vi "DrivePath.vi"() -> ()   [LabVIEW 2018]
uses:
  Dawgma Programming Library/Controls/PurePursuit/PathFileData.ctl
  Dawgma Programming Library/Controls/PurePursuit/RobotNeededPathData.ctl
  Framework/Robot Global Data.vi
panel:
  in  "NoWait":bool
  in  "Index":i32
  in  "Path":string
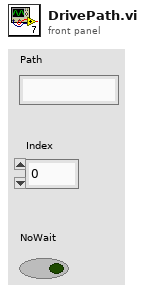
[diagram p1: front panel]
types:
  T1 = typedef "PathFileData.ctl" = cluster{"RobotNeeded":T2, "Meta":cluster{"Path (px)":cluster{i32, i32}[], "RobotWidth":dbl, "RobotLength":dbl, "CenterOfRotYOffset":dbl, "Roundedness":dbl, "StartingPositionPreset":u32}}
  T2 = typedef "RobotNeededPathData.ctl" = cluster{"Path":cluster{dbl, dbl}[], "MaxVel":dbl, "MaxAccel":dbl, "Backwards?":bool, "PointSpacing":dbl, "LookaheadDist":dbl, "Speed/Curve":dbl, "SlowDistanceAtEnd":dbl, "SlowSpeed":dbl, "MaxDeAccel":dbl}
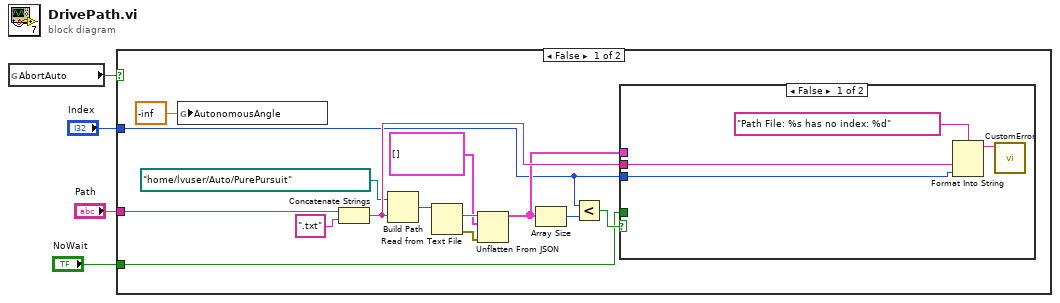
[diagram p0: block diagram]
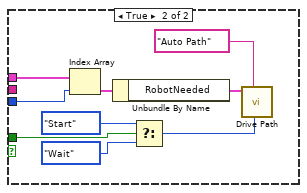
[diagram p2: hidden frame]
diagram:
  n1 = global read "Robot Global Data.vi" "AbortAuto"() -> (w4:bool)
  n2 = case shown="False" w4 {
    tunnel: "Index" -> [w7 _]
    tunnel: "NoWait" -> [w6 _]
    tunnel: "Path" -> [w5 _]
    frame False {
      n3 = global write "Robot Global Data.vi" "AutonomousAngle"(-inf ("AutonomousAngle")) -> ()
      n4 = Concatenate Strings(w5, ".txt" ("string")) -> (w18:string)
      n5 = Build Path(base path=path "/home/lvuser/Auto/PurePursuit", name or relative path=w18) -> (appended path=w14:path)
      n6 = Read from Text File(file (use dialog)=w14) -> (text=w13:string, error out=w12:errorcluster)  [unwired: 3 in, 2 out]
      n7 = Unflatten From JSON(JSON string=w13, type and defaults=T1[] [], error in (no error)=w12) -> (value=w15:T1[])  [unwired: 4 in, 1 out]
      n8 = Array Size(array=w15) -> (size(s)=w16:i32)
      n9 = Less?(x=w7, y=w16) -> (x < y?=w17:bool)
      n10 = case shown="False" w17 {
        tunnel: w7 -> [w20 w31]
        tunnel: w6 -> [_ w27]
        tunnel: w15 -> [_ w23]
        tunnel: w18 -> [w19 _]
        frame False {
          n11 = Format Into String(format string="Path File: %s has no index: %d", w19, w20) -> (resulting string=w22:string)  [unwired: 2 in, 1 out]
          n12 = call "CustomError.vi"("String"=w22) -> ()  [unwired: 10 in, 1 out]
        }
        frame True {
          n13 = Index Array(array=w23, index=w31) -> (element=w30:T1)
          n14 = Unbundle By Name(w30) -> ("RobotNeeded"=w29:T2)
          n15 = Select(t=enum16{"Start", "Wait"}."Start" ("Synchronication"), s=w27, f=enum16{"Start", "Wait"}."Wait" ("Synchronication")) -> (s? t:f=w24:enum16{"Start", "Wait"})
          n16 = call "Drive Path.vi"("Synchronication"=w24, "Description"="Auto Path", "Path"=w29) -> ()  [unwired: 8 in, 1 out]
        }
      }
    }
    frame True {
    }
  }
